vi "System Explorer - Add content to System Explorer library.vi"(8 "error in (no error)":errorcluster, 9 "Extra Page Names":string[](array[string]), 10 "Project Root":path, 11 "CD Wizard - Internal Data":T1) -> (0 "error out":errorcluster, 1 "Extra Page VIs":path[](array[path]), 2 "System Explorer Main VI":path, 3 "Load Help File VI":path)   [LabVIEW 2020, in "NIVS_Consolidated_CDW_MetaDataObj.lvclass"]
doc: "Add all virtual folders and VIs to the System Explorer library."
uses:
  NIVS_Consolidated_CDW_MetaDataObj.lvclass
  Internal data.ctl
  CD System Explorer lvlib.ctl
  Add Item - Type.ctl
  CD System Explorer lvlib.vi
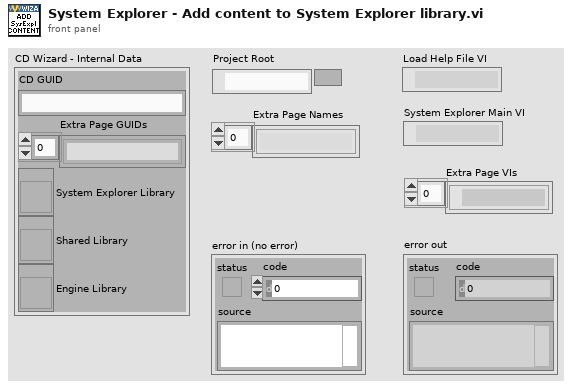
[diagram p1: front panel]
types:
  T1 = typedef "NIVS_Consolidated_CDW_MetaDataObj.lvclass/Internal data.ctl" = cluster{"CD GUID":string, "Extra Page GUIDs":string[], "System Explorer Library":refnum<vi>, "Shared Library":refnum<vi>, "Engine Library":refnum<vi>}
  T2 = typedef "NIVS_Consolidated_CDW_MetaDataObj.lvclass/CD System Explorer lvlib.ctl" = enum16{"LibraryFileName", "LibraryFolderName", "System Explorer.FolderName", "System Explorer.Dynamically Called.FolderName", "System Explorer.Dynamically Called.Extra Pages.FolderName", "System Explorer.Dynamically Called.Extra Pages.TemplatePathAndName", "System Explorer.Dynamically Called.Main Page.VIName", "System Explorer.Dynamically Called.Main Page.TemplatePathAndName", "System Explorer.Dynamically Called.Initialization VI.VIName", "System Explorer.Dynamically Called.Initialization VI.TemplatePathAndName", "System Explorer.SubVI.FolderName", "System Explorer.Types.FolderName", "System Explorer.ActionVIOnCompile.VIName", "System Explorer.ExportConfigRTM.VIName", "System Explorer.PPL.ExportConfigRTM.VIName", "System Explorer.LoadHelpFile.VIName", "System Explorer.PPL.LoadHelpFile.VIName", "System Explorer.SetRTDriverVIsFilePaths.VIName", "System Explorer.ClearRTDriverVIs.VIName"}
  T3 = typedef "NIVS_Consolidated_CDW_MetaDataObj.lvclass/Add Item - Type.ctl" = string
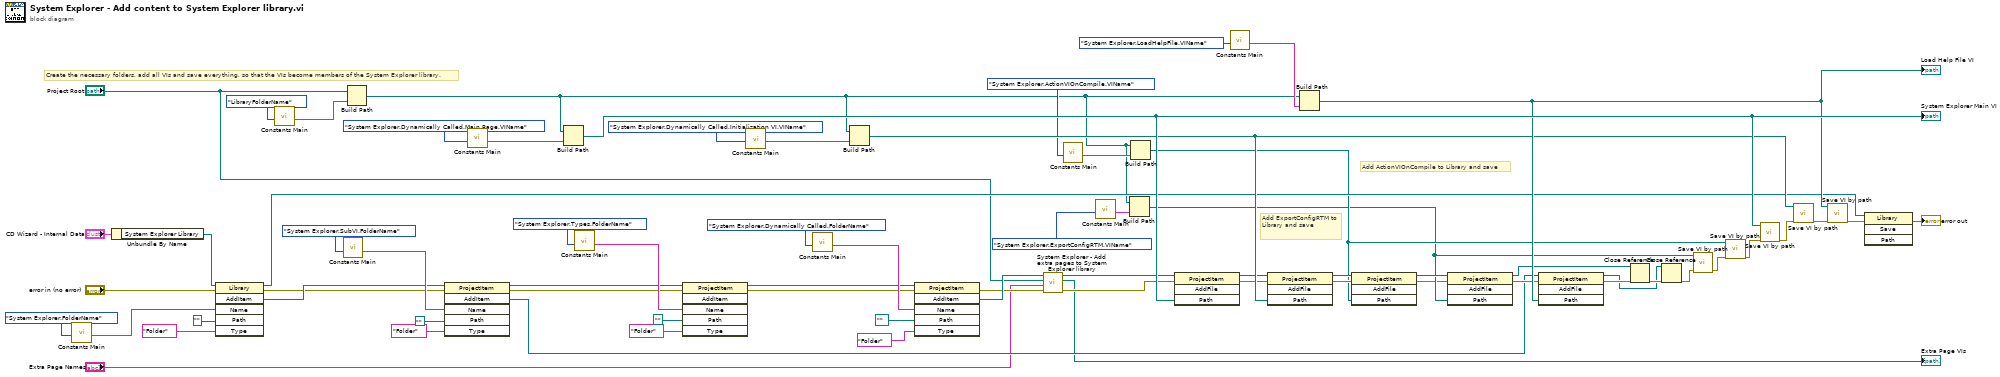
[diagram p0: block diagram]
diagram:
  # "Create the necessary folders, add all VIs and save everything, so that the VIs become members of the System Explorer library."
  # "Add ExportConfigRTM to Library and save"
  # "Add ActionVIOnCompile to Library and save"
  n1 = call-poly "Constants Main.vi"("Action"=CD_System_Explorer_lvlib."System Explorer.FolderName") -> ("Output"=w63:string)  [unwired: 10 in]
  n2 = Unbundle By Name("CD Wizard - Internal Data") -> ("System Explorer Library"=w38:refnum<vi>)
  n3 = invoke class="Library" method="AddItem"(reference=w38, error in="error in (no error)", "Name"=w63, "Path"=path "", "Type"=T3 "Folder" ("Add Item - Type")) -> (reference out=w40:refnum<vi>, error out=w7:errorcluster, "AddItem"=w39:refnum<vi>)  [unwired: 1 in, 3 out]
  n4 = call-poly "Constants Main.vi"("Action"=CD_System_Explorer_lvlib."LibraryFolderName") -> ("Output"=w33:string)  [unwired: 10 in]
  n5 = call-poly "Constants Main.vi"("Action"=CD_System_Explorer_lvlib."System Explorer.SubVI.FolderName") -> ("Output"=w55:string)  [unwired: 10 in]
  n6 = Build Path(base path="Project Root", name or relative path=w33) -> (appended path=w11:path)
  n7 = invoke class="ProjectItem" method="AddItem"(reference=w39, error in=w7, "Name"=w55, "Path"=path "", "Type"=T3 "Folder" ("Add Item - Type")) -> (reference out=w42:refnum<vi>, error out=w6:errorcluster, "AddItem"=w13:refnum<vi>)  [unwired: 1 in, 3 out]
  n8 = call-poly "Constants Main.vi"("Action"=CD_System_Explorer_lvlib."System Explorer.Dynamically Called.Main Page.VIName") -> ("Output"=w61:string)  [unwired: 10 in]
  n9 = Build Path(base path=w11, name or relative path=w61) -> (appended path=w68:path)
  "System Explorer Main VI" <- w68
  n10 = call-poly "Constants Main.vi"("Action"=CD_System_Explorer_lvlib."System Explorer.Types.FolderName") -> ("Output"=w50:string)  [unwired: 10 in]
  n11 = invoke class="ProjectItem" method="AddItem"(reference=w42, error in=w6, "Name"=w50, "Path"=path "", "Type"=T3 "Folder" ("Add Item - Type")) -> (reference out=w41:refnum<vi>, error out=w5:errorcluster)  [unwired: 1 in, 4 out]
  n12 = call-poly "Constants Main.vi"("Action"=CD_System_Explorer_lvlib."System Explorer.Dynamically Called.Initialization VI.VIName") -> ("Output"=w60:string)  [unwired: 10 in]
  n13 = call-poly "Constants Main.vi"("Action"=CD_System_Explorer_lvlib."System Explorer.Dynamically Called.FolderName") -> ("Output"=w45:string)  [unwired: 10 in]
  n14 = Build Path(base path=w11, name or relative path=w60) -> (appended path=w57:path)
  n15 = invoke class="ProjectItem" method="AddItem"(reference=w41, error in=w5, "Name"=w45, "Path"=path "", "Type"=T3 "Folder" ("Add Item - Type")) -> (error out=w35:errorcluster, "AddItem"=w37:refnum<vi>)  [unwired: 1 in, 4 out]
  n16 = call "System Explorer - Add extra pages to System Explorer library.vi"("error in (no error)"=w35, "Extra Page Names"="Extra Page Names", "Project Root"="Project Root", "ProjectItem in"=w37) -> ("error out"=w4:errorcluster, "Extra Page VIs"=→"Extra Page VIs":path[], "ProjectItem out"=w36:refnum<vi>)  [unwired: 5 in]
  n17 = call-poly "Constants Main.vi"("Action"=CD_System_Explorer_lvlib."System Explorer.ActionVIOnCompile.VIName") -> ("Output"=w27:string)  [unwired: 10 in]
  n18 = call-poly "Constants Main.vi"("Action"=CD_System_Explorer_lvlib."System Explorer.ExportConfigRTM.VIName") -> ("Output"=w21:string)  [unwired: 10 in]
  n19 = Build Path(base path=w11, name or relative path=w21) -> (appended path=w20:path)
  n20 = Build Path(base path=w11, name or relative path=w27) -> (appended path=w29:path)
  n21 = invoke class="ProjectItem" method="AddFile"(reference=w36, error in=w4, "Path"=w68) -> (reference out=w43:refnum<vi>, error out=w44:errorcluster)  [unwired: 1 in, 2 out]
  n22 = call-poly "Constants Main.vi"("Action"=CD_System_Explorer_lvlib."System Explorer.LoadHelpFile.VIName") -> ("Output"=w12:string)  [unwired: 10 in]
  n23 = invoke class="ProjectItem" method="AddFile"(reference=w43, error in=w44, "Path"=w57) -> (reference out=w32:refnum<vi>, error out=w31:errorcluster)  [unwired: 1 in, 2 out]
  n24 = Build Path(base path=w11, name or relative path=w12) -> (appended path=w67:path)
  "Load Help File VI" <- w67
  n25 = invoke class="ProjectItem" method="AddFile"(reference=w32, error in=w31, "Path"=w29) -> (reference out=w26:refnum<vi>, error out=w17:errorcluster)  [unwired: 1 in, 2 out]
  n26 = invoke class="ProjectItem" method="AddFile"(reference=w26, error in=w17, "Path"=w20) -> (reference out=w16:refnum<vi>, error out=w25:errorcluster)  [unwired: 1 in, 2 out]
  n27 = invoke class="ProjectItem" method="AddFile"(reference=w13, error in=w25, "Path"=w67) -> (reference out=w14:refnum<vi>, error out=w19:errorcluster)  [unwired: 1 in, 2 out]
  n28 = Close Reference(reference=w16, error in (no error)=w19) -> (error out=w23:errorcluster)
  n29 = Close Reference(reference=w14, error in (no error)=w23) -> (error out=w15:errorcluster)
  n30 = call "Save VI by path.vi"("error in (no error)"=w15, "VI path"=w20) -> ("error out"=w24:errorcluster)  [unwired: 9 in]
  n31 = call "Save VI by path.vi"("error in (no error)"=w24, "VI path"=w29) -> ("error out"=w30:errorcluster)  [unwired: 9 in]
  n32 = call "Save VI by path.vi"("error in (no error)"=w30, "VI path"=w68) -> ("error out"=w58:errorcluster)  [unwired: 9 in]
  n33 = call "Save VI by path.vi"("error in (no error)"=w58, "VI path"=w57) -> ("error out"=w10:errorcluster)  [unwired: 9 in]
  n34 = call "Save VI by path.vi"("error in (no error)"=w10, "VI path"=w67) -> ("error out"=w9:errorcluster)  [unwired: 9 in]
  n35 = invoke class="Library" method="Save"(reference=w40, error in=w9) -> (error out=→"error out":errorcluster)  [unwired: 2 in, 3 out]
